vi "DSF.Engine.Framework.Set Engine Base Pointer.vi"(8 "error in (no error)":errorcluster, 9 "engine size":u64, 10 "engine base address":u64 format="%.0x", 11 "Framework in":refnum<class "DSF.Engine.Framework.lvclass">) -> (0 "error out":errorcluster, 3 "Framework out":refnum<class "DSF.Engine.Framework.lvclass">)   [LabVIEW 2017, in "DSF.Engine.lvlib" / "DSF.Engine.Framework.lvclass"]
uses:
  DSF.Engine.Framework.lvclass
  Pointer/DSF.Engine.Pointer.DBL.lvclass
  DSF.Engine.Framework.lvclass/DSF.Engine.Framework.ctl
  Plugin/DSF.Engine.Plugin.lvclass
  Built/PharLap x86/Dependencies/c/Memory Manager.lvlibp/1abvi3w/vi.lib/National Instruments/Memory Manager/Classes/Pointer/Memory.Pointer.lvclass
  C:/Git/DSF/DSF Core/Built/Windows/Dependencies/Memory Manager.lvlibp/1abvi3w/vi.lib/National Instruments/Memory Manager/Classes/Pointer/Memory.Pointer.lvclass
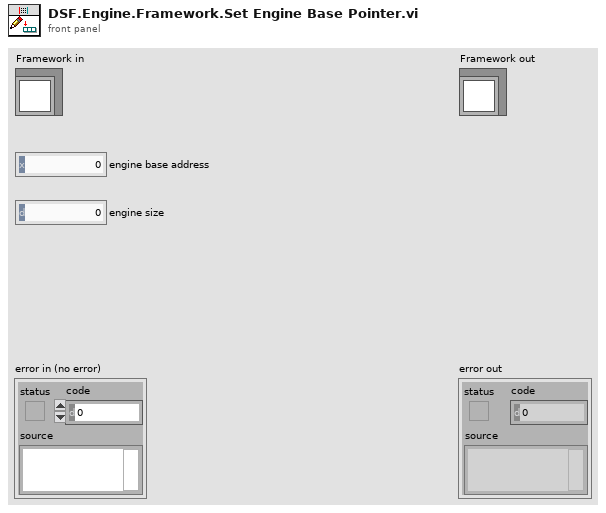
[diagram p1: front panel]
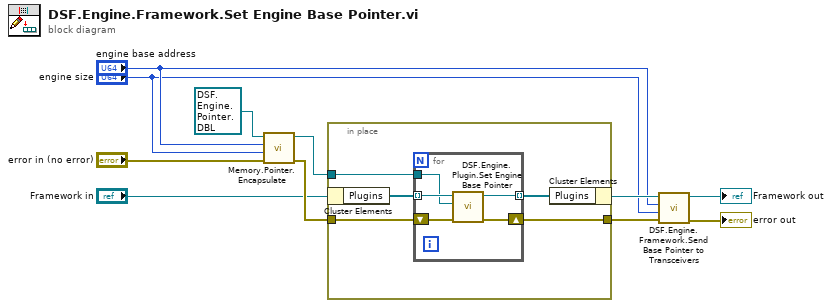
[diagram p0: block diagram]
diagram:
  n1 = call "Memory.Pointer.Encapsulate.vi"("error in (no error)"="error in (no error)", "size"="engine size", "address"="engine base address", "Pointer type"=refnum<class "DSF.Engine.Pointer.DBL.lvclass"> refnum ("DSF.Engine.lvlib:DBL Pointer")) -> ("error out"=w9:errorcluster, "Pointer out"=w8:refnum<class "DSF.Engine.Pointer.DBL.lvclass">)  [unwired: 6 in]
  n2 = in-place {
    in-place-border: w9 -> [w13]
    in-place-border: [w14] -> w6
    in-place-border: w8 -> [w12]
    n3 = in-place-cluster #1("Framework in") -> ("Plugins"=w16:refnum<class "DSF.Engine.Plugin.lvclass">[])
    n4 = for {
      tunnel: w16 -> [w21] mode=indexing
      tunnel: [w20] -> w15 mode=indexing
      shift-right: [w19] -> w14
      shift-left: w13 -> [w18]
      tunnel: w12 -> [w17]
      n5 = call "DSF.Engine.Plugin.Set Engine Base Pointer.vi"("error in (no error)"=w18, "Engine Base Pointer"=w17, "Plugin in"=w21) -> ("error out"=w19:errorcluster, "Plugin out"=w20:refnum<class "DSF.Engine.Plugin.lvclass">)  [unwired: 7 in]
    }
    n6 = in-place-cluster #1("Plugins"=w15) -> (w7:refnum<class "DSF.Engine.Framework.lvclass">)
  }
  n7 = call "DSF.Engine.Framework.Send Base Pointer to Transceivers.vi"("error in (no error)"=w6, "engine size"="engine size", "engine base address"="engine base address", "Framework in"=w7) -> ("error out"=→"error out":errorcluster, "Framework out"=→"Framework out":refnum<class "DSF.Engine.Framework.lvclass">)  [unwired: 6 in]
